vi "Read Indicator.vi"(9 "Control in":refnum<class "Control.lvclass">) -> (3 "Control out":refnum<class "Control.lvclass">, 4 "Indicator":bool)   [LabVIEW 2014, in "Raspberry Pi Compatible Compiler for LabVIEW.lvlib" / "Control.lvclass"]
uses:
  Control.lvclass
  Control.lvclass/Control.ctl
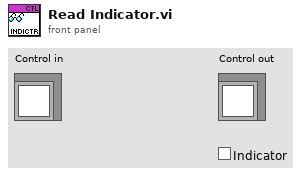
[diagram p1: front panel]
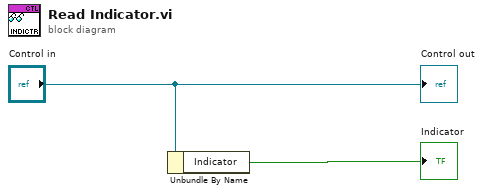
[diagram p0: block diagram]
diagram:
  n1 = Unbundle By Name("Control in") -> ("Indicator"=→"Indicator":bool)
  "Control out" <- "Control in"
